vi "readSettings.vi"(7 "name":string, 8 "error in":errorcluster, 9 "log":string, 10 "parameter table":string[][](array[string]), 11 "DeviceInterface in":refnum<class "DeviceInterface.lvclass">) -> (0 "error out":errorcluster, 1 "log out":string, 2 "parameter table out":string[][](array[string]), 3 "DeviceInterface out":refnum<class "DeviceInterface.lvclass">)   [LabVIEW 2013, in "EMV-Test.lvlib"]
uses:
  lib/EMV-Test.lvlib
  DeviceInterface/DeviceInterface.lvclass
  <vilib>/regexp/Match Regular Expression.xnode
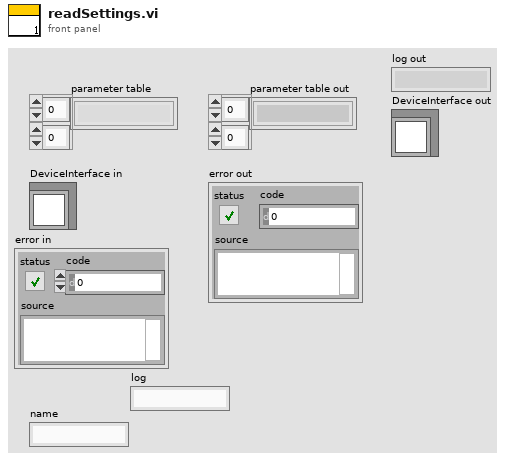
[diagram p1: front panel]
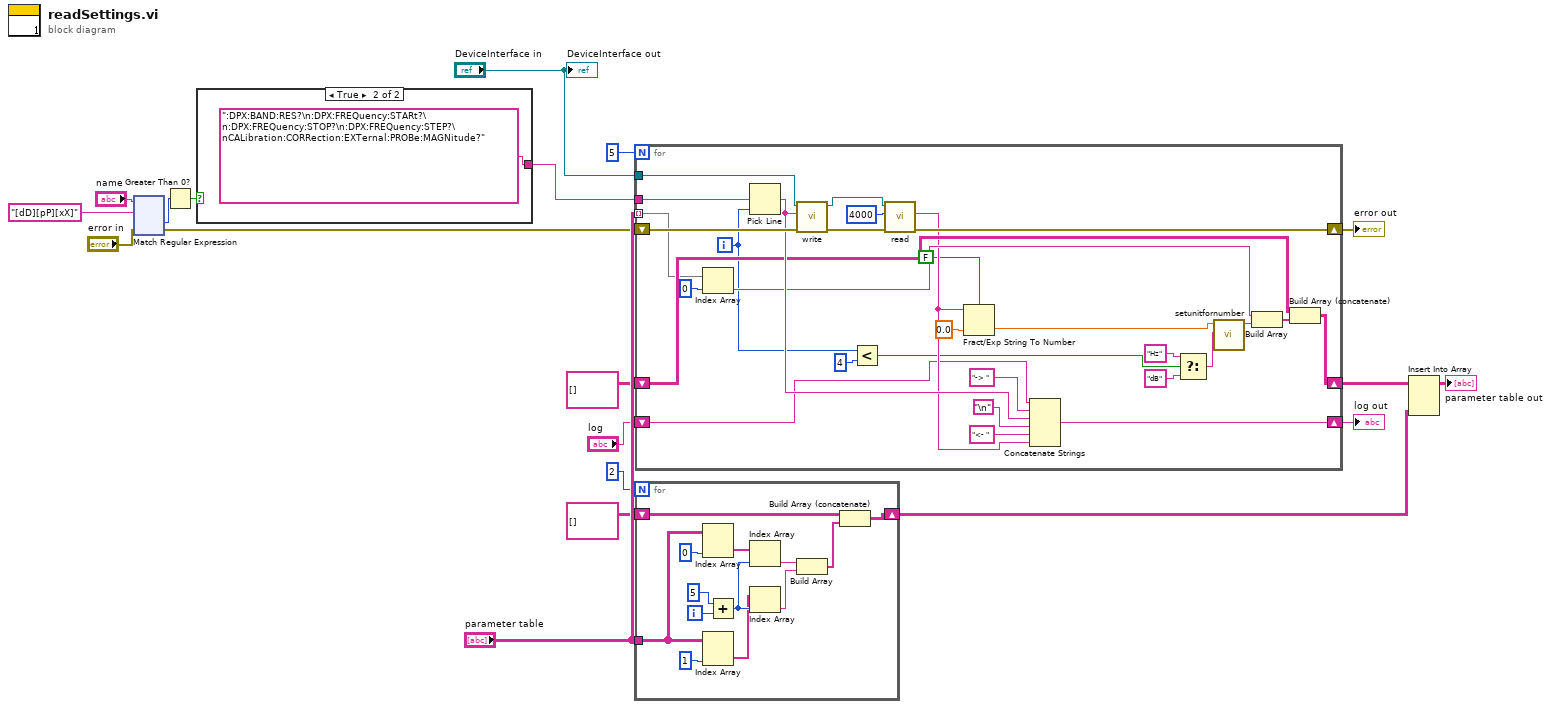
[diagram p0: block diagram]
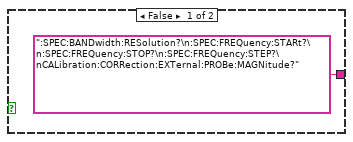
[diagram p2: hidden frame]
diagram:
  n1 = xnode "Match Regular Expression"("input string"="name", "regular expression"="[dD][pP][xX]", "error in"="error in") -> ("offset past match"=w9:i32, "error out"=w5:errorcluster)  [unwired: 3 in, 3 out]
  n2 = Greater Than 0?(x=w9) -> (x > 0?=w3:bool)
  n3 = case shown="True" w3 {
    tunnel: [":SPEC:BANDwidth:RESolution?\n:SPEC:FREQuency:STARt?\n:SPEC:FREQuency:STOP?\n:SPEC:FREQuency:STEP?\nCALibration:CORRection:EXTernal:PROBe:MAGNitude?" ("string") ":DPX:BAND:RES?\n:DPX:FREQuency:STARt?\n:DPX:FREQuency:STOP?\n:DPX:FREQuency:STEP?\nCALibration:CORRection:EXTernal:PROBe:MAGNitude?" ("string")] -> w10
    frame False {
    }
    frame True {
    }
  }
  n4 = for {
    N: 5 -> [_]
    tunnel: w10 -> [w43]
    tunnel: "DeviceInterface in" -> [w50]
    shift-right: [w44] -> w18
    shift-left: w5 -> [w49]
    shift-right: [w36] -> w13
    shift-left: string[][] [] -> [w41]
    tunnel: "parameter table" -> [w39] mode=indexing
    shift-right: [w32] -> w1
    shift-left: "log" -> [w31]
    i -> [w26]
    n5 = Index Array(array=w39, index=0) -> (element=w37:string)
    n6 = Pick Line(multi-line string=w43, line index=w26) -> (output string=w42:string)  [unwired: 1 in]
    n7 = call-dynamic "write.vi"("error in (no error)"=w49, "String to send"=w42, "DeviceInterface in"=w50) -> ("error out"=w51:errorcluster, "DeviceInterface out"=w48:refnum<class "DeviceInterface.lvclass">)  [unwired: 7 in]
    n8 = Less?(x=w26, y=4) -> (x < y?=w27:bool)
    n9 = call-dynamic "read.vi"("error in (no error)"=w51, "timeout (ms)"=4000, "DeviceInterface in"=w48) -> ("error out"=w44:errorcluster, "Return String"=w34:string)  [unwired: 6 in, 1 out]
    n10 = Fract/Exp String To Number(use system decimal point (T)=FALSE, string=w34, default (0 dbl)=0.0) -> (number=w22:dbl)  [unwired: 1 in, 1 out]
    n11 = Concatenate Strings(w31, "-> " ("string"), w42, "\n", "<- " ("string"), w34) -> (w32:string)
    n12 = Select(t="Hz", s=w27, f="dB") -> (s? t:f=w24:string)
    n13 = call "setunitfornumber.vi"("Einheit"=w24, "Numeric"=w22) -> ("String"=w30:string)  [unwired: 9 in]
    n14 = Build Array(w37, w30) -> (w40:string[])
    n15 = Build Array (concatenate)(w41, w40) -> (w36:string[][])
  }
  "error out" <- w18
  "log out" <- w1
  n16 = for {
    N: 2 -> [_]
    tunnel: "parameter table" -> [w52]
    shift-right: [w61] -> w14
    shift-left: string[][] [] -> [w60]
    i -> [w64]
    n17 = Index Array(array=w52, index (col)=0 ("disabled index (col)")) -> (element=w62:string[])  [unwired: 1 in]
    n18 = Index Array(array=w52, index (col)=1 ("disabled index (col)")) -> (element=w54:string[])  [unwired: 1 in]
    n19 = Add(x=5, y=w64) -> (x+y=w55:i32)
    n20 = Index Array(array=w62, index=w55) -> (element=w59:string)
    n21 = Index Array(array=w54, index=w55) -> (element=w53:string)
    n22 = Build Array(w59, w53) -> (w58:string[])
    n23 = Build Array (concatenate)(w60, w58) -> (w61:string[][])
  }
  n24 = Insert Into Array(array=w13, new element=w14) -> (→"parameter table out":string[][])  [unwired: 2 in]
  "DeviceInterface out" <- "DeviceInterface in"
